vi "Image Generator.vi"(6 "ColorRamp in":refnum<vi>, 7 "Lithography Data":T2(array[cluster]), 8 "error in (no error)":errorcluster, 9 "Resolution":i32=444, 11 "Image Reference In":T3) -> (0 "error out":errorcluster, 3 "Image Reference Out":T3(plugin-control))   [LabVIEW 2016]
doc: "This VI generates a rendered image given the lithography data."
uses:
  <vilib>/vision/Image Controls.llb/IMAQ Image.ctl
  <userlib>/LevyLab/Relay Box/Type_defs/Resistor--enum.ctl
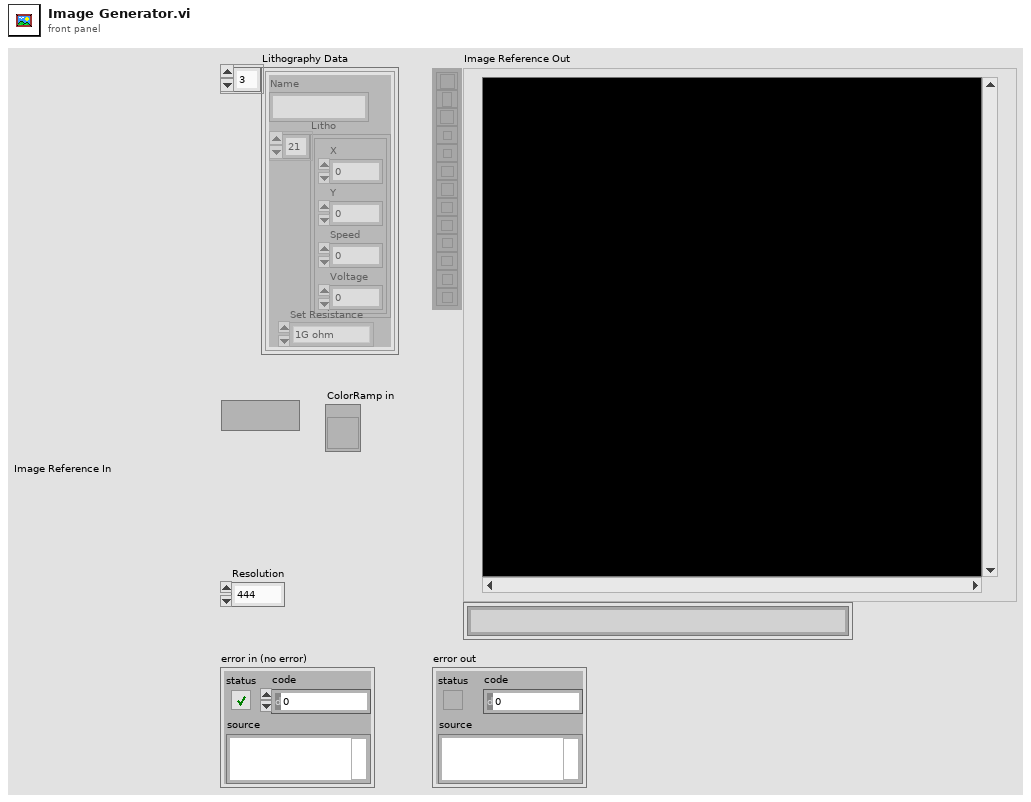
[diagram p1: front panel]
types:
  T1 = typedef "Resistor--enum.ctl" = enum16{"open", "discharge tip", "0 ohms", "100k ohm", "10M ohm", "1G ohm"}
  T2 = cluster{"Name":string, "Litho":cluster{"X":dbl, "Y":dbl, "Speed":dbl, "Voltage":dbl}[], "Set Resistance":T1}[]
  T3 = typedef "IMAQ Image.ctl" = refnum<image>
  T4 = cluster{"X":dbl, "Y":dbl, "Speed":dbl, "Voltage":dbl}[]
  T5 = cluster{"X":dbl, "Y":dbl, "Speed":dbl, "Voltage":dbl}
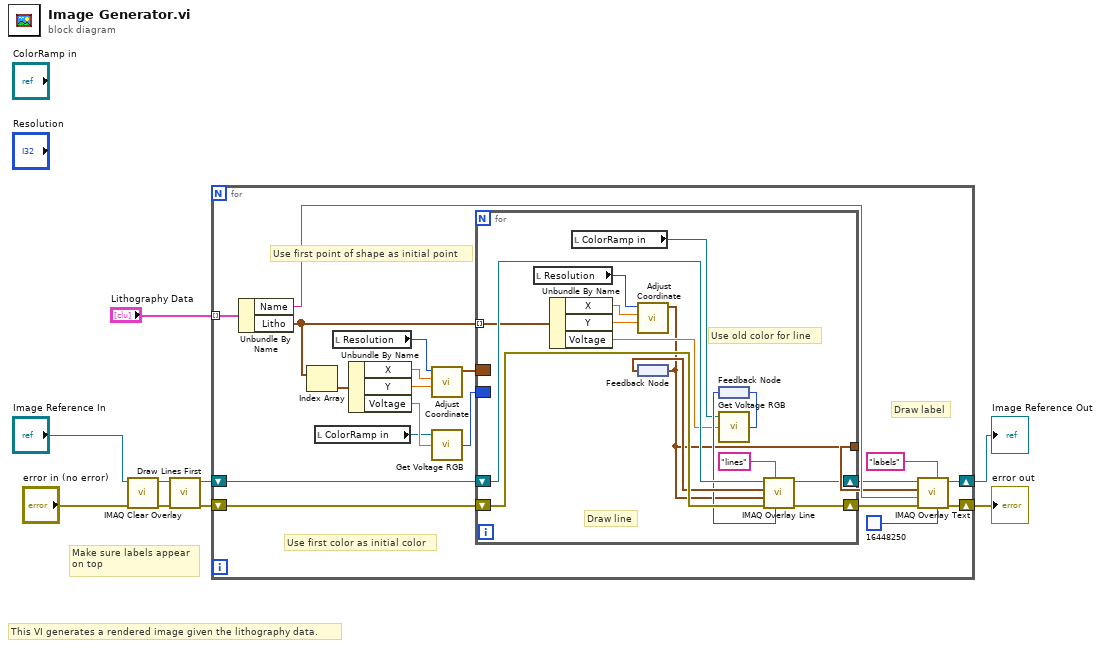
[diagram p0: block diagram]
diagram:
  # "This VI generates a rendered image given the lithography data."
  # "Make sure labels appear\non top"
  n1 = call "IMAQ Clear Overlay"("error in (no error)"="error in (no error)", "Image"="Image Reference In") -> ("error out"=w1:errorcluster, "Image Out"=w4:T3)  [unwired: 8 in]
  n2 = call "Draw Lines First.vi"("error in (no error)"=w1, "Refnum in"=w4) -> ("error out"=w5:errorcluster, "Refnum out"=w6:T3)  [unwired: 8 in]
  n3 = for {
    tunnel: "Lithography Data" -> [w21] mode=indexing
    shift-right: [w22] -> w8
    shift-left: w6 -> [w28]
    shift-right: [w24] -> w7
    shift-left: w5 -> [w29]
    # "Draw label"
    # "Use first color as initial color"
    # "Use first point of shape as initial point"
    n4 = Unbundle By Name(w21) -> ("Name"=w27:string, "Litho"=w19:T4)
    n5 = Index Array(array=w19) -> (element=w18:T5)  [unwired: 1 in]
    n6 = local read "ColorRamp in"() -> (w14:refnum<vi>)
    n7 = local read "Resolution"() -> (w10:i32)
    n8 = Unbundle By Name(w18) -> ("X"=w13:dbl, "Y"=w12:dbl, "Voltage"=w16:dbl)
    n9 = call "Adjust Coordinate.vi"("Y"=w12, "X"=w13, "Resolution"=w10) -> ("Adjusted Coordinate"=w11:cluster{dbl, dbl})  [unwired: 7 in, 1 out]
    n10 = call "Get Voltage RGB.vi"("Voltage"=w16, "ColorRamp in"=w14) -> ("RGB Value"=w15:u32)  [unwired: 1 in, 2 out]
    n11 = for {
      tunnel: w19 -> [w40] mode=indexing
      shift-right: [w43] -> w23
      shift-left: w28 -> [w44]
      shift-right: [w41] -> w25
      shift-left: w29 -> [w42]
      tunnel: [w30] -> w20
      border: w11 -> [_]
      border: w15 -> [_]
      # "Draw line"
      # "Use old color for line"
      n12 = local read "Resolution"() -> (w33:i32)
      n13 = Unbundle By Name(w40) -> ("X"=w32:dbl, "Y"=w31:dbl, "Voltage"=w34:dbl)
      n14 = local read "ColorRamp in"() -> (w35:refnum<vi>)
      n15 = call "Adjust Coordinate.vi"("Y"=w31, "X"=w32, "Resolution"=w33) -> ("Adjusted Coordinate"=w30:cluster{dbl, dbl})  [unwired: 7 in, 1 out]
      n16 = feedback-in #1(w30) -> ()
      n17 = feedback #1() -> (w39:cluster{dbl, dbl})
      n18 = feedback #2() -> (w37:u32)
      n19 = call "Get Voltage RGB.vi"("Voltage"=w34, "ColorRamp in"=w35) -> ("RGB Value"=w36:u32)  [unwired: 1 in, 2 out]
      n20 = feedback-in #2(w36) -> ()
      n21 = call "IMAQ Overlay Line"("Color"=w37, "Group"="lines", "error in (no error)"=w42, "End Point"=w30, "Start Point"=w39, "Image"=w44) -> ("error out"=w41:errorcluster, "Image Out"=w43:T3)  [unwired: 4 in]
    }
    n22 = call "IMAQ Overlay Text"("BG Color (Transparent)"=u32 16448250, "Group"="labels", "error in (no error)"=w25, "String"=w27, "Origin"=w20, "Image"=w23) -> ("error out"=w24:errorcluster, "Image Out"=w22:T3)  [unwired: 4 in]
  }
  "Image Reference Out" <- w8
  "error out" <- w7
